vi "DQMH_API_CleanUp.vi"(11 "error in (no error)":errorcluster) -> (15 "error out":errorcluster)   [LabVIEW 2016, in "DQMH_API.lvclass"]
uses:
  <resource>/Framework/Providers/Open_GDS/UML/DQMH_API_class/DQMH_API.lvclass
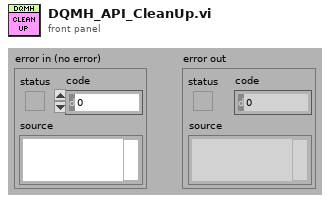
[diagram p1: front panel]
types:
  T1 = typedef "DQMH_API.lvclass/ObjectAttributes.ctl" = cluster{"Get Module Type Info":refnum<vi>, "Script New Module":refnum<vi>, "Script New Event":refnum<vi>}
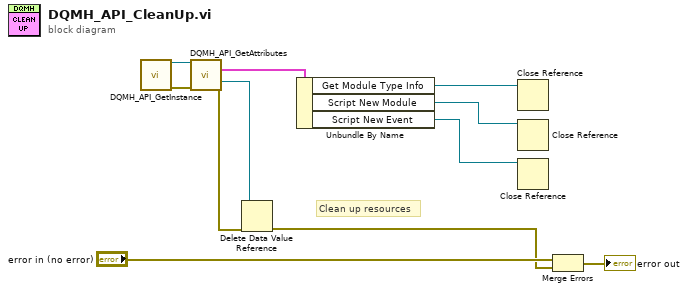
[diagram p0: block diagram]
diagram:
  # "Clean up resources"
  n1 = call <resource>:"DQMH_API_GetInstance.vi"() -> ("reference out"=w8:refnum<class "DQMH_API.lvclass">, "error out"=w9:errorcluster)  [unwired: 11 in, 3 out]
  n2 = call <resource>:"DQMH_API_GetAttributes.vi"("reference in"=w8, "error in (no error)"=w9) -> ("Data"=w10:T1, "DataRef"=w6:refnum<data-value>, "error out"=w7:errorcluster)  [unwired: 10 in, 1 out]
  n3 = Delete Data Value Reference(data value reference=w6, error in=w7) -> (error out=w4:errorcluster)  [unwired: 1 out]
  n4 = Unbundle By Name(w10) -> ("Get Module Type Info"=w3:refnum<vi>, "Script New Module"=w2:refnum<vi>, "Script New Event"=w1:refnum<vi>)
  n5 = Close Reference(reference=w3) -> ()  [unwired: 1 in, 1 out]
  n6 = Close Reference(reference=w2) -> ()  [unwired: 1 in, 1 out]
  n7 = Close Reference(reference=w1) -> ()  [unwired: 1 in, 1 out]
  n8 = Merge Errors("error in (no error)", w4) -> (→"error out":errorcluster)
